vi "Read Blackboard.vi"(8 "error in (no error)":errorcluster, 11 "Blackboard_Boolean in":refnum<class "Blackboard_String.lvclass">) -> (0 "error out":errorcluster, 2 "Blackboard.lvclass":refnum<class "Blackboard.lvclass">, 3 "Blackboard_Boolean out":refnum<class "Blackboard_String.lvclass">)   [LabVIEW 2021, in "Blackboard_String.lvclass"]
uses:
  Blackboard_String.lvclass
  Blackboard.lvclass
  Blackboard_String.lvclass/Blackboard_String.ctl
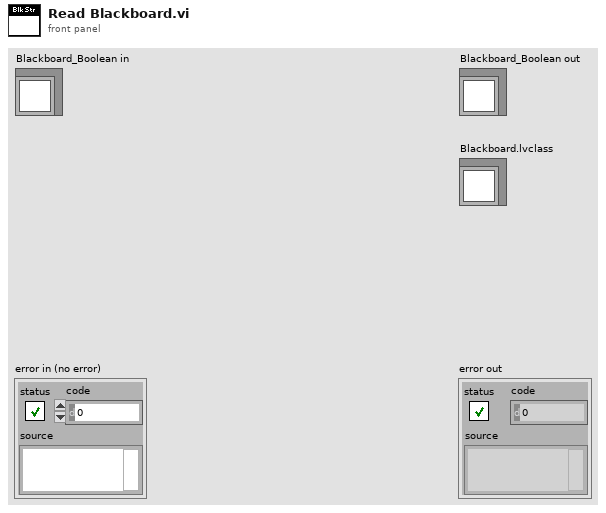
[diagram p1: front panel]
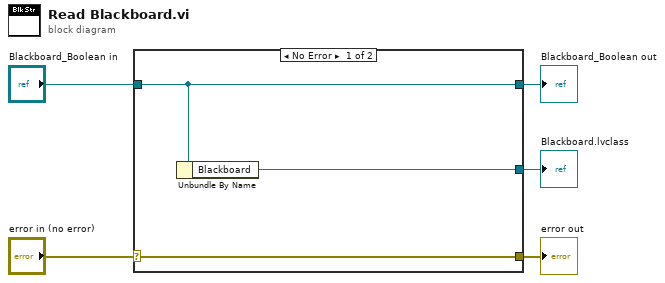
[diagram p0: block diagram]
diagram:
  n1 = case shown="No Error" "error in (no error)" {
    selector: "error in (no error)" -> [w8 w9]
    tunnel: [w8 w9] -> w4
    tunnel: [w7 w10] -> w2
    tunnel: "Blackboard_Boolean in" -> [w7 w10]
    tunnel: [w6 _] -> w1
    frame No Error {
      n2 = Unbundle By Name(w7) -> ("Blackboard"=w6:refnum<class "Blackboard.lvclass">)
    }
    frame Error {
    }
  }
  "error out" <- w4
  "Blackboard_Boolean out" <- w2
  "Blackboard.lvclass" <- w1
